vi "capacidade.vi"() -> ()   [LabVIEW 2016]
panel:
  in  "stop":bool
  in  "CC Value":dbl caption="current (0.0)"
  in  "Current Enable":bool
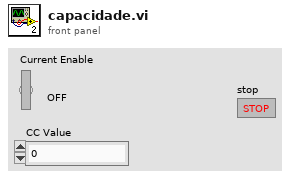
[diagram p1: front panel]
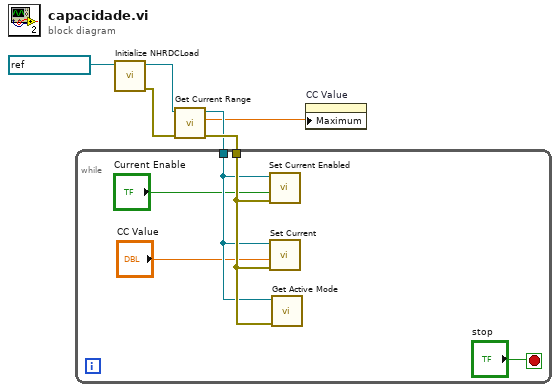
[diagram p0: block diagram]
diagram:
  n1 = call <instrlib>:"Initialize NHRDCLoad.vi"("resource name"=refnum<visa-resource-name> "DC Load 1") -> ("error out"=w4:errorcluster, "instrument handle out"=w5:refnum<visa-resource-name>)  [unwired: 9 in]
  n2 = call <instrlib>:"Get Current Range.vi"("error in (no error)"=w4, "instrument handle"=w5) -> ("error out"=w3:errorcluster, "current range"=w1:dbl, "instrument handle out"=w2:refnum<visa-resource-name>)  [unwired: 7 in]
  n3 = while {
    tunnel: w3 -> [w11]
    tunnel: w2 -> [w10]
    stop <- "stop" stop-if-true
    n4 = call <instrlib>:"Set Current Enabled.vi"("error in (no error)"=w11, "current enabled (false)"="Current Enable", "instrument handle"=w10) -> ()  [unwired: 7 in, 2 out]
    n5 = call <instrlib>:"Set Current.vi"("error in (no error)"=w11, "current (0.0)"="CC Value", "instrument handle"=w10) -> ()  [unwired: 7 in, 2 out]
    n6 = call <instrlib>:"Get Active Mode.vi"("error in (no error)"=w11, "instrument handle"=w10) -> ()  [unwired: 7 in, 3 out]
  }
  n7 = property on="CC Value" class="DigNum (strict)"("Maximum"=w1) -> ()  [unwired: 2 in, 2 out]
